vi "Amplitude_Simulation.vi"(11 "Sim Scope Operation":T1) -> (3 "Amplitude":dbl)   [LabVIEW 2011, in "Simulated Scope.lvclass"]
uses:
  Simulated Scope.lvclass
  Simulated Scope Operation.ctl
panel:
  out "Count":dbl
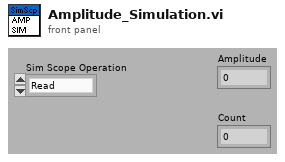
[diagram p1: front panel]
types:
  T1 = typedef "Simulated Scope.lvclass/Simulated Scope Operation.ctl" = enum16{"Read", "Clear"}
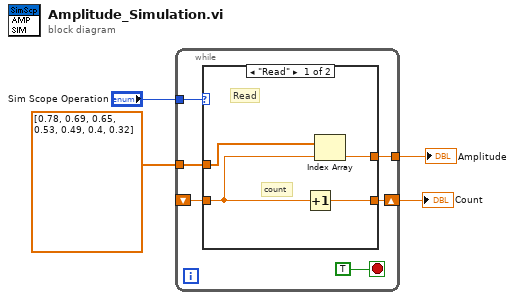
[diagram p0: block diagram]
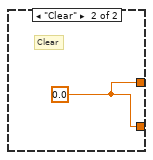
[diagram p2: hidden frame]
diagram:
  n1 = while {
    tunnel: "Sim Scope Operation" -> [w9]
    shift-right: [w8] -> w3
    shift-left: _ -> [w7]
    tunnel: dbl[] [0.78, 0.69, 0.65, 0.53, 0.49, 0.4, 0.32] ("Freq Amp Array") -> [w6]
    tunnel: [w5] -> w4
    stop <- TRUE stop-if-true
    n2 = case shown="\"Read\"" w9 {
      tunnel: [w14 w15] -> w8
      tunnel: w7 -> [w12 _]
      tunnel: w6 -> [w13 _]
      tunnel: [w11 w15] -> w5
      frame "Read" {
        # "count"
        # "Read"
        n3 = Increment(x=w12) -> (x+1=w14:dbl)
        n4 = Index Array(array=w13, index=w12) -> (element=w11:dbl)
      }
      frame "Clear" {
        w15 = 0.0 ("Amplitude")
        # "Clear"
      }
    }
  }
  "Amplitude" <- w4
  "Count" <- w3
